vi "ADC Data capture and Process Original.vi"(0 "ADC Output Read Method":T2(ring)=enum."Read .dat file", 1 "Select the Tab to project":T1(ring)=enum."ADC Sine", 2 "ADC Input":enum16{"Sine Wave", "Ramp / Triangle"}(ring), 3 "No.of samples(SNR)":i32=4096, 4 "Resolution":i32=12, 5 "active edge":i32(ring)=10280, 6 "Inputs for Dyanmic para":T9={"Fundamental Frequency"=100000.0, "Sampling Frequncy"=3999610.0, "No of Harmonics"=9, "Window"=enum."7 Term B-Harris", "Blackman (fundamental power) bins)"=1.0}, 7 "Samples per Channel":i32=4096 caption="No.of Samples(capture)", 8 "Oversampling":bool, 9 "Oversampling ratio":i32, 10 "Drop LSB":bool, 11 "Save data":T15, 12 "Waveform":i64[](array[numeric]), 13 "Path to Read":path=path "C/Users/a0230227/Desktop/save.dat", 14 "Start & Stop Bit":cluster{"Start":i32, "Stop":i32}={"Start"=40, "Stop"=4055}, 15 "length":i32=4096, 17 "Set_Freq":dbl=100017.0, 24 "path to save":T14={"Path to Save plot"=path "D/Tenor_176P/DYN_PAR_C004/DAT/D001_TEMPP30C_VDD1.2_VDDA3.3_16B_SE_ADCA__vicA_aggX_PLT_CAP_200821_1740_33.jpg", "Path to Raw Data plot"=path "D/Tenor_176P/DYN_PAR_C004/DAT/D001_TEMPP30C_VDD1.2_VDDA3.3_16B_SE_ADCA__vicA_aggX_RAW_DAT_200821_1740_33.csv"}) -> (18 "Min Max":T4, 19 "detected Throughput":dbl, 20 "output cluster":T7, 21 "Dynamic Parameters":T8, 22 "max code":ext, 23 "min code":ext, 25 "Valid Capture":bool)   [LabVIEW 2021] (continued)
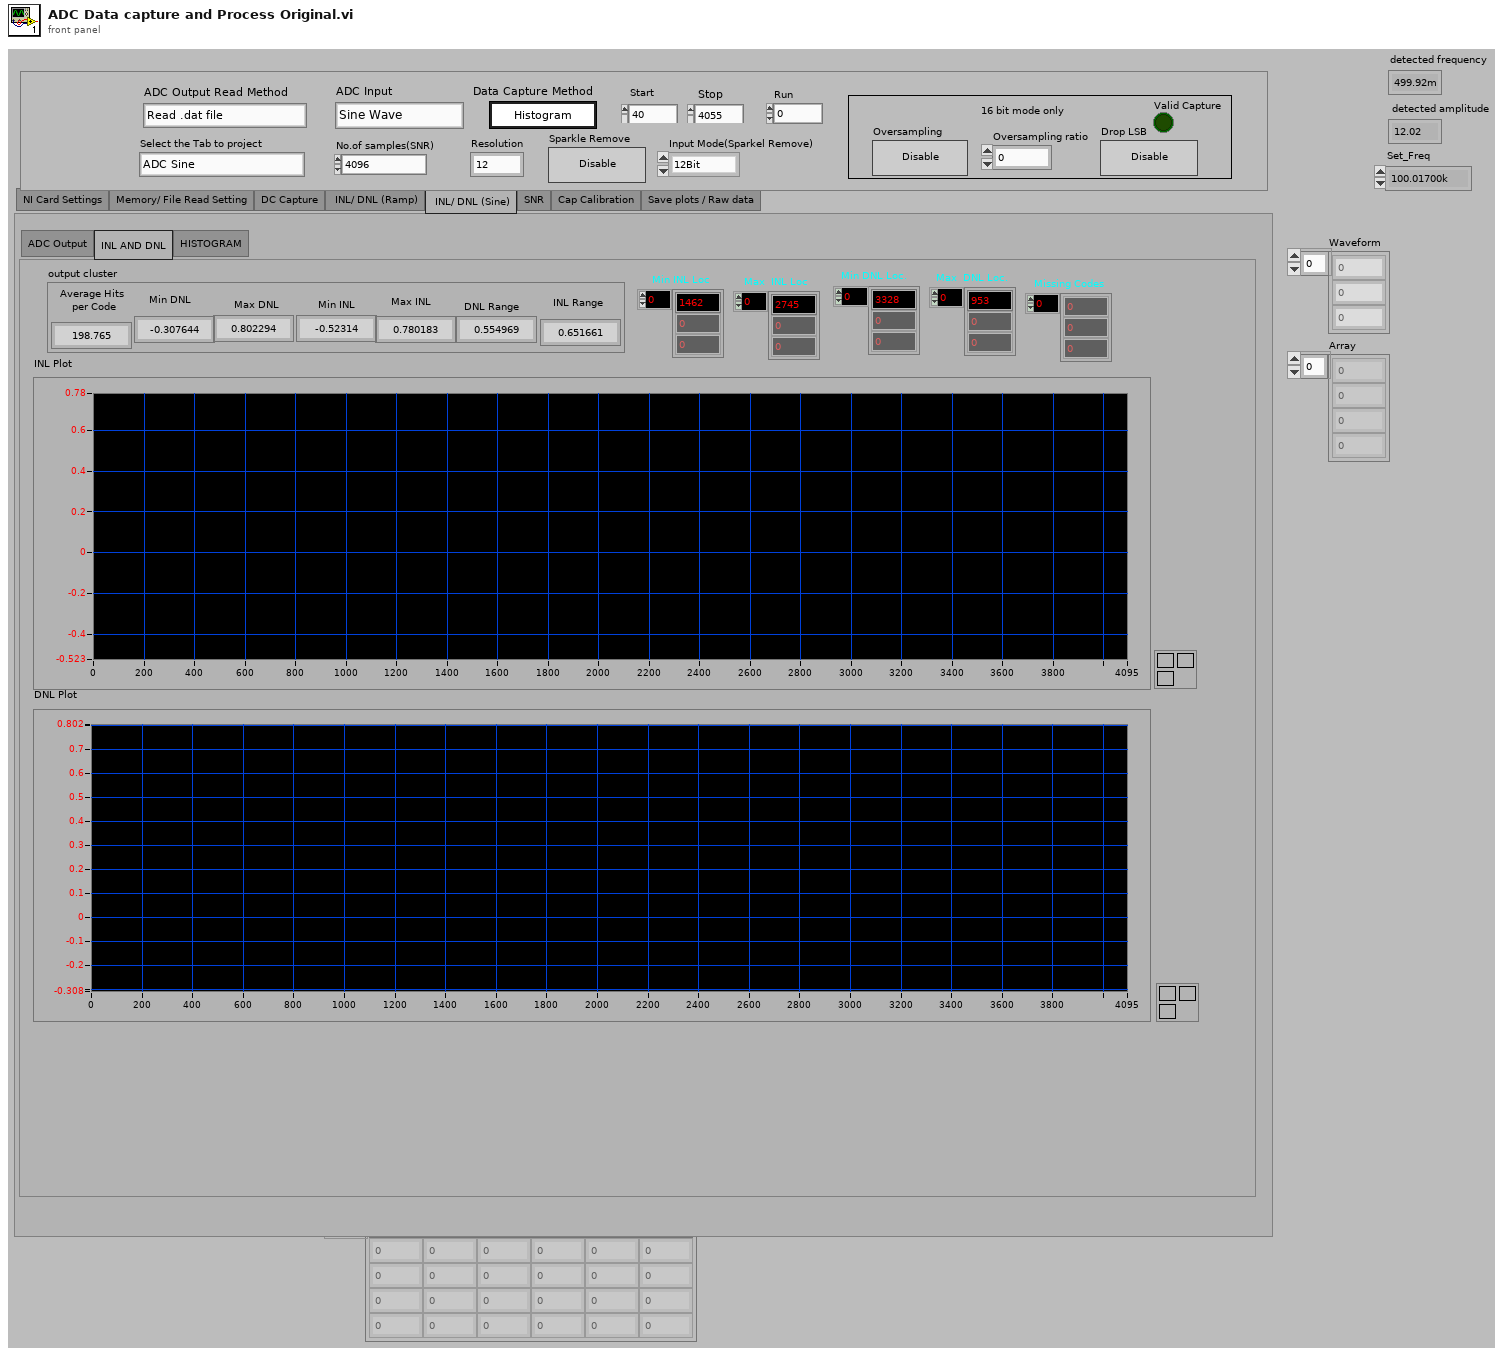
[diagram p1: front panel]
types:
  T1 = enum32{"NI Card Settings", "Memory Read Setting", "DC Capture", "ADC Ramp", "ADC Sine", "SNR", "Cap Calibration"}
  T2 = enum32{"Read from Memory", "Read .dat file", "NI Card Capture", "None"}
  T3 = enum32{"NI Card Settings", "Memory/ File Read Setting", "DC Capture", " INL/ DNL (Ramp)", " INL/ DNL (Sine)", "SNR", "Cap Calibration", "Save plots / Raw data"}
  T4 = cluster{"Min":dbl, "Max":dbl, "delta":dbl, "Average Code":dbl, "Standard Deviation":dbl}
  T5 = cluster{"Min INL":dbl, "Max INL":dbl, "Min DNL":dbl, "Max DNL":dbl, "INL Range":dbl, "DNL Range":dbl, "Avg Hits/Code":dbl}
  T6 = enum32{"ADC Output", "TRIMMED DATA", "INL AND DNL", "HISTOGRAM"}
  T7 = cluster{"Average Hits \nper Code ":dbl, "Min DNL":dbl, "Min INL":dbl, "Max INL":dbl, "Max DNL":dbl, "DNL Range":dbl, "INL Range":dbl}
  T8 = cluster{"SNR":dbl, "SNRD":dbl, "THD":dbl, "ENOB (SNRD)":dbl, "SFDR":dbl, "ENOB (SNR)":dbl, "Noise Power":dbl, "Signal power":dbl}
  T9 = cluster{"Fundamental Frequency":dbl, "Sampling Frequncy":dbl, "No of Harmonics":u8, "Window":enum16{"None ", "Hanning", "Hamming", "Blackman-Harris", "Exact Blackman", "Blackman", "Flat Top", "4 Term B-Harris ", "7 Term B-Harris"}, "Blackman (fundamental power) bins)":dbl}
  T10 = enum32{"ADC Output", "FFT Magnitude plot", " FFT plot"}
  T11 = cluster{"Ideal Power Bin":dbl, "Actual Power Bin":dbl, "Signal Strength (dB)":dbl}
  T12 = cluster{"ADC Reference(V)":dbl, "Bin Width":dbl, "PSRR/ CMRR  ":bool}
  T13 = cluster{"Fundamental Frequnecy (Calculated)":dbl, "Harmonic Frequencies":dbl[], "Harmonic Amplitudes":dbl[]}
  T14 = cluster{"Path to Save plot":path, "Path to Raw Data plot":path}
  T15 = cluster{"Save INL/DNL Plot(Ramp)":bool, "Save SNR Plot":bool, "Save INL/DNL Plot(Sine)":bool, "Save INL/DNL Raw Data(Ramp)":bool, "Save SNR Raw Data":bool, "Save INL/DNL Raw Data(Sine)":bool, "Save DC Raw data":bool, "Save  Raw Data(Sine)":bool}
  T16 = enum16{"Initialize", "Read output", "Post process", "Cap Calib", "Save data", "Exit"}
  T17 = cluster{"Average Hits \nper Code ":dbl, "Min\nDNL":dbl, dbl, dbl, "Max\nDNL":dbl, dbl, dbl}
  T18 = enum16{"None ", "Hanning", "Hamming", "Blackman-Harris", "Exact Blackman", "Blackman", "Flat Top", "4 Term B-Harris ", "7 Term B-Harris"}
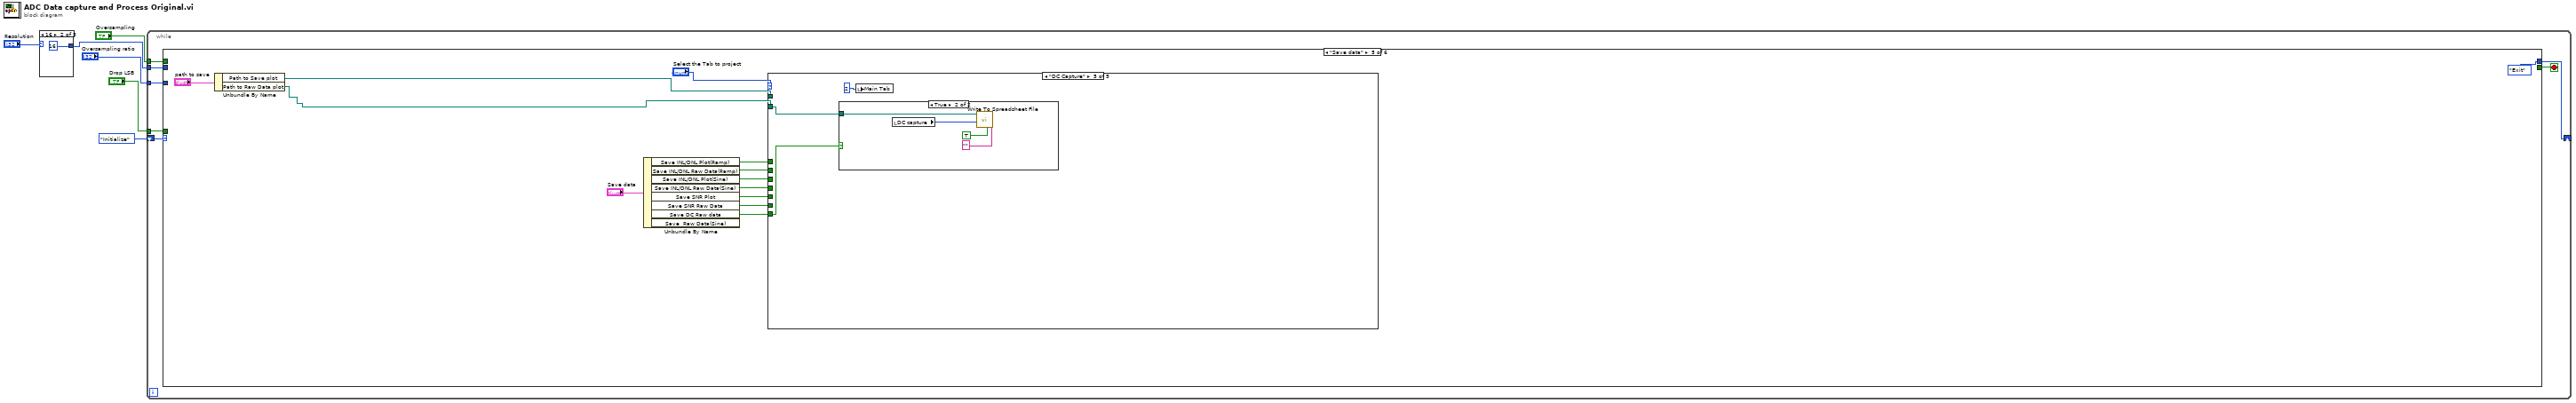
[diagram p0: block diagram]
diagram:
  n1 = case shown="16" "Resolution" {
    tunnel: [18 16 14 12 10] -> w5
    frame 18 {
    }
    frame 16 {
    }
    frame 14, Default {
    }
    frame 12 {
    }
    frame 10 {
    }
  }
  n2 = while {
    shift-right: [w17] -> _
    shift-left: T16."Initialize" -> [w18]
    tunnel: w5 -> [w15]
    tunnel: "Oversampling" -> [w14]
    tunnel: "Drop LSB" -> [w13]
    tunnel: "Oversampling ratio" -> [w12]
    stop <- w16 stop-if-true
    n3 = case shown="\"Save data\"" w18 {
      tunnel: [T16."Read output" w41 w104 T16."Save data" T16."Exit" _] -> w17
      tunnel: [_ _ _ _ _ TRUE] -> w16
      tunnel: w15 -> [_ _ w111 _ _ _]
      tunnel: w14 -> [_ _ w101 _ _ _]
      tunnel: w13 -> [_ _ w103 _ _ _]
      tunnel: w12 -> [_ _ w102 _ _ _]
      frame "Initialize", Default {
        n4 = local read "No.of samples(SNR)"() -> (w19:i32)
        n5 = local write "Samples per Channel"(w19) -> ()
      }
      frame "Read output" {
        w26 = waveform(i64) {"t0"=timestamp(0 s since 1904-01-01), "dt"=1.0, "Y"=[]}  # waveform
        n6 = case shown="\"NI Card Capture\", Default" "ADC Output Read Method" {
          tunnel: [w51 _ w70 "Waveform"] -> w27
          tunnel: [T16."Post process" _ T16."Post process" T16."Post process"] -> w41
          frame "Read .dat file" {
            w50 = 0  # index
            w56 = 8192 ("index")
            w61 = 1 ("index")
            n7 = call-poly <vilib>:"Read From Spreadsheet File.vi"("delimiter (\\t)"="Delimiter (\\t)", "file path (dialog if empty)"="Path to Read") -> ("all rows"=w63:i64[][])  [unwired: 5 in, 4 out]
            n8 = Index Array(array=w63, index (col)=0 ("disabled index (col)")) -> (element=w54:i64[])  [unwired: 1 in]
            n9 = Split 1D Array(array=w54, index=w61) -> (second subarray=w52:i64[])  [unwired: 1 out]
            n10 = Multiply(x=w56, y=1) -> (x*y=w59:i32)
            n11 = Multiply(x=2 ("y"), y=w56) -> (x*y=w57:i32)
            n12 = Multiply(x=w56, y=3) -> ()  [unwired: 1 out]
            n13 = Array Subset(array=w52, index=w61, length=w56) -> ()  [unwired: 1 out]
            n14 = Array Subset(array=w52, index=w59, length=w56) -> ()  [unwired: 1 out]
            n15 = Array Subset(array=w52, index=w57, length=w56) -> ()  [unwired: 1 out]
            n16 = Array Subset(array=w52, index=w50, length="length") -> (w51:i64[])
          }
          frame "None" {
          }
          frame "NI Card Capture", Default {
            n17 = case shown="\"Ramp / Triangle\"" "ADC Input" {
              tunnel: "Port" -> [w87 w98]
              tunnel: "Source" -> [w86 w97]
              tunnel: "Rate" -> [w85 w96]
              tunnel: "Timeout" -> [w84 w95]
              tunnel: [_ w93] -> w69
              tunnel: [w80 w94] -> w70
              tunnel: "No.of samples(SNR)" -> [w83 w92]
              tunnel: "Samples per Channel" -> [w81 w91]
              tunnel: "Sparkle Remove" -> [w79 _]
              tunnel: "active edge" -> [w78 w89]
              frame "Sine Wave", Default {
                n18 = call "DATA_CAPTURE_SNR.vi"("Port"=w87, "Source"=w86, "No. of samples to process"=w83, "Samples per Channel"=w81, "Rate"=w85, "active edge"=w78, "timeout"=w84, "Histogram Capture Method SNR"=w79, "NI card Cont/Single Capture"=FALSE ("Histogram Capture Method SNR")) -> ("Waveform"=w80:u32[])  [unwired: 5 in, 5 out]
              }
              frame "Ramp / Triangle" {
                n19 = call "DATA_CAPTURE_SNR.vi"("Port"=w98, "Source"=w97, "No. of samples to process"=w92, "Samples per Channel"=w91, "Rate"=w96, "active edge"=w89, "timeout"=w95, "Histogram Capture Method SNR"=FALSE, "NI card Cont/Single Capture"=FALSE ("Histogram Capture Method SNR")) -> ("Waveform"=w94:u32[], "Trimmed Wave"=w93:u32[])  [unwired: 5 in, 4 out]
              }
            }
            "Trimmed Wave" <- w69
          }
          frame "Read from Memory" {
          }
        }
        "Ramp Waveform" <- w27
        "Sine Waveform" <- w27
        "Read Data from Device" <- w27
        "Captured Data" <- w27
        "DC capture" <- w27
        n20 = Bundle By Name(cluster=w26, "Y"=w27) -> (w25:waveform(i64))
        n21 = Array Size(array=w27) -> (size(s)=w37:i32)
        n22 = Array Max & Min(array=w27) -> (max value=→"max code":i64, min value=→"min code":i64)  [unwired: 2 out]
        n23 = Decrement(x=w37) -> (x-1=w36:i32)
        n24 = call-poly <vilib>:"Extract Single Tone Information.vi"("time signal in"=w25) -> ("detected amplitude"=→"detected amplitude":dbl, "detected frequency"=w22:dbl)  [unwired: 5 in, 4 out]
        "detected frequency" <- w22
        n25 = for {
          N: w36 -> [_]
          tunnel: w27 -> [w48]
          tunnel: [w42] -> w34 mode=indexing
          i -> [w46]
          n26 = Increment(x=w46) -> (x+1=w47:i32)
          n27 = Index Array(array=w48, index=w46) -> (element=w44:i64)
          n28 = Index Array(array=w48, index=w47) -> (element=w45:i64)
          n29 = Subtract(x=w45, y=w44) -> (x-y=w43:i64)
          n30 = Absolute Value(x=w43) -> (abs(x)=w42:i64)
        }
        n31 = Divide(x="Set_Freq", y=w22) -> (x/y=→"detected Throughput":dbl)
        n32 = Add Array Elements(numeric array=w34) -> (sum=w32:i64)
        n33 = Array Max & Min(array=w34) -> (max value=w29:i64)  [unwired: 3 out]
        n34 = Array Size(array=w34) -> (size(s)=w31:i32)
        n35 = Divide(x=w32, y=w31) -> (x/y=w33:dbl)
        n36 = Multiply(x=2.0, y=w33) -> (x*y=w28:dbl)
        n37 = Less?(x=w29, y=w28) -> (x < y?=→"Valid Capture":bool)
      }
      frame "Post process" {
        n38 = local read "Select the Tab to project"() -> (w117:T1)
        n39 = local read "Read Data from Device"() -> (w108:dbl[])
        n40 = local read "No.of samples(SNR)"() -> (w110:i32)
        n41 = Equal?(x=w117, y=T1."Cap Calibration" ("Select the Tab to project")) -> (x = y?=w118:bool)
        n42 = Unbundle By Name("Start & Stop Bit") -> ("Start"=w113:i32, "Stop"=w112:i32)
        n43 = Select(t=T1."ADC Sine" ("Select the Tab to project"), s=w118, f=w117) -> (s? t:f=w116:T1)
        n44 = case shown="\"DC Capture\", Default" w116 {
          tunnel: w108 -> [w123 w239 w311 w376]
          tunnel: "Data Capture Method" -> [w120 w237 w344 _]
          tunnel: w113 -> [_ w236 w343 _]
          tunnel: w112 -> [_ w235 w342 _]
          tunnel: w111 -> [_ w238 w341 w375]
          tunnel: w110 -> [_ _ _ w377]
          tunnel: [_ w234 w329 _] -> w109
          tunnel: [T16."Save data" T16."Save data" T16."Cap Calib" T16."Save data"] -> w104
          tunnel: w101 -> [_ _ w308 w373]
          tunnel: w103 -> [_ _ w307 w372]
          tunnel: w102 -> [_ _ w309 w371]
          frame "DC Capture", Default {
            n45 = property on="Raw Data CH2" class="Arr (strict)"("Visible"="CH Swtich (To see other CH O/P)") -> ()  [unwired: 2 in, 2 out]
            n46 = property on="Standard Deviation (CH2)" class="DigNum (strict)"("Visible"="CH Swtich (To see other CH O/P)") -> ()  [unwired: 2 in, 2 out]
            n47 = property on="Raw Data CH1" class="Arr (strict)"("Visible"="CH Swtich (To see other CH O/P)") -> ()  [unwired: 2 in, 2 out]
            n48 = property on="Average Code (CH2)" class="DigNum (strict)"("Visible"="CH Swtich (To see other CH O/P)") -> ()  [unwired: 2 in, 2 out]
            n49 = case shown="False" w120 {
              tunnel: w123 -> [w126 w194]
              tunnel: "CH Swtich (To see other CH O/P)" -> [w125 _]
              tunnel: [w124 w180] -> w119
              frame False {
                n50 = case shown="True" w125 {
                  tunnel: w126 -> [w131 w168]
                  tunnel: [w127 w160] -> w124
                  frame True {
                    w137 = 10 ("index")
                    w150 = 10 ("index")
                    n51 = Decimate 1D Array(w131) -> (w147:dbl[], w138:dbl[])
                    "Raw Data CH2" <- w147
                    "Raw Data CH1" <- w138
                    n52 = Split 1D Array(array=w147, index=w150) -> (second subarray=w149:dbl[])  [unwired: 1 out]
                    n53 = Split 1D Array(array=w138, index=w137) -> (second subarray=w146:dbl[])  [unwired: 1 out]
                    n54 = Array Size(array=w149) -> (size(s)=w151:i32)
                    n55 = Array Size(array=w146) -> (size(s)=w145:i32)
                    n56 = Subtract(x=w151, y=w150) -> (x-y=w154:i32)
                    n57 = Subtract(x=w145, y=w137) -> (x-y=w135:i32)
                    n58 = Split 1D Array(array=w149, index=w154) -> (first subarray=w153:dbl[])  [unwired: 1 out]
                    n59 = Split 1D Array(array=w146, index=w135) -> (first subarray=w143:dbl[])  [unwired: 1 out]
                    n60 = Array Size(array=w153) -> (size(s)=w152:i32)
                    n61 = Array Size(array=w143) -> (size(s)=w144:i32)
                    n62 = To Double Precision Float(number=w153) -> (double precision float=w155:dbl[])
                    n63 = To Double Precision Float(number=w143) -> (double precision float=w134:dbl[])
                    n64 = Add Array Elements(numeric array=w155) -> (sum=w159:dbl)
                    n65 = Add Array Elements(numeric array=w134) -> (sum=w139:dbl)
                    n66 = Divide(x=w159, y=w152) -> (x/y=w132:dbl)
                    "Average Code (CH2)" <- w132
                    n67 = Divide(x=w139, y=w144) -> (x/y=w129:dbl)
                    n68 = Subtract(x=w155, y=w132) -> (x-y=w158:dbl[])
                    n69 = Subtract(x=w134, y=w129) -> (x-y=w140:dbl[])
                    n70 = Square(x=w158) -> (x^2=w157:dbl[])
                    n71 = Square(x=w140) -> (x^2=w141:dbl[])
                    n72 = Add Array Elements(numeric array=w157) -> (sum=w156:dbl)
                    n73 = Add Array Elements(numeric array=w141) -> (sum=w142:dbl)
                    n74 = Divide(x=w156, y=w152) -> (x/y=w148:dbl)
                    n75 = Divide(x=w142, y=w144) -> (x/y=w136:dbl)
                    n76 = Square Root(x=w148) -> (sqrt(x)=→"Standard Deviation (CH2)":dbl)
                    n77 = Square Root(x=w136) -> (sqrt(x)=w128:dbl)
                    n78 = local read "Min Max"() -> (w130:T4)
                    n79 = Bundle By Name(cluster=w130, "Average Code"=w129, "Standard Deviation"=w128) -> (w127:T4)
                  }
                  frame False {
                    w172 = 10 ("index")
                    n80 = Split 1D Array(array=w168, index=w172) -> (second subarray=w179:dbl[])  [unwired: 1 out]
                    n81 = Array Size(array=w179) -> (size(s)=w178:i32)
                    n82 = Subtract(x=w178, y=w172) -> (x-y=w170:i32)
                    n83 = Split 1D Array(array=w179, index=w170) -> (first subarray=w167:dbl[])  [unwired: 1 out]
                    n84 = Array Size(array=w167) -> (size(s)=w177:i32)
                    n85 = To Double Precision Float(number=w167) -> (double precision float=w169:dbl[])
                    n86 = Add Array Elements(numeric array=w169) -> (sum=w173:dbl)
                    n87 = Divide(x=w173, y=w177) -> (x/y=w162:dbl)
                    n88 = Subtract(x=w169, y=w162) -> (x-y=w174:dbl[])
                    n89 = Square(x=w174) -> (x^2=w175:dbl[])
                    n90 = Add Array Elements(numeric array=w175) -> (sum=w176:dbl)
                    n91 = Divide(x=w176, y=w177) -> (x/y=w171:dbl)
                    n92 = Array Max & Min(array=w167) -> (max value=w164:dbl, min value=w163:dbl)  [unwired: 2 out]
                    n93 = local read "Min Max"() -> (w166:T4)
                    n94 = Subtract(x=w164, y=w163) -> (x-y=w165:dbl)
                    n95 = Square Root(x=w171) -> (sqrt(x)=w161:dbl)
                    n96 = Bundle By Name(cluster=w166, "Standard Deviation"=w161, "Average Code"=w162, "Max"=w164, "Min"=w163, "delta"=w165) -> (w160:T4)
                  }
                }
              }
              frame True {
                n97 = for {
                  tunnel: w194 -> [w227] mode=indexing
                  shift-right: [w231] -> w203
                  shift-left: 0.0 ("x*y") -> [w232]
                  tunnel: w194 -> [w230]
                  tunnel: [w229] -> w202
                  shift-right: [w218] -> _
                  shift-left: TRUE ("x != 0?") -> [w225]
                  shift-right: [w221] -> w185
                  shift-left: i32[] [] -> [w222]
                  i -> [w224]
                  n98 = Add Array Elements(numeric array=w230) -> (sum=w229:dbl)
                  n99 = Not Equal To 0?(x=w227) -> (x != 0?=w226:bool)
                  n100 = Multiply(x=w227, y=w224) -> (x*y=w228:dbl)
                  n101 = Build Array (concatenate)(w222, w224) -> (w223:i32[])
                  n102 = And(x=w225, y=w226) -> (x .and. y?=w220:bool)
                  n103 = Add(x=w232, y=w228) -> (x+y=w231:dbl)
                  n104 = Select(t=w223, s=w220, f=w222) -> (s? t:f=w221:i32[])
                  n105 = Select(t=FALSE ("x != 0?"), s=w220, f=TRUE ("x != 0?")) -> (s? t:f=w218:bool)
                }
                n106 = Divide(x=w203, y=w202) -> (x/y=w181:dbl)
                n107 = Array Size(array=w185) -> (size(s)=w183:i32)
                n108 = Index Array(array=w185, index=0) -> (element=w186:i32)
                n109 = Split 1D Array(array=w194, index=w186) -> (second subarray=w189:dbl[])  [unwired: 1 out]
                n110 = Subtract(x=w183, y=15 ("x")) -> (x-y=w182:i32)
                n111 = Array Max & Min(array=w189) -> (max index (indices)=w197:i32)  [unwired: 3 out]
                n112 = Greater?(x=w197, y=w182) -> (0:w198:bool)
                n113 = case shown="True" w198 {
                  tunnel: w197 -> [w206 w213]
                  tunnel: [w205 w213] -> w193
                  tunnel: 10 ("y") -> [w210 w212]
                  tunnel: w189 -> [w209 w216]
                  tunnel: [w206 w215] -> w192
                  tunnel: [_ w211] -> w187
                  frame True {
                    n114 = Subtract(x=w206, y=w210) -> (x-y=w207:i32)
                    n115 = Split 1D Array(array=w209, index=w207) -> (first subarray=w208:dbl[])  [unwired: 1 out]
                    n116 = Array Max & Min(array=w208) -> (max index (indices)=w205:i32)  [unwired: 3 out]
                  }
                  frame False {
                    n117 = Add(x=w213, y=w212) -> (x+y=w211:i32)
                    n118 = Split 1D Array(array=w216, index=w211) -> (second subarray=w214:dbl[])  [unwired: 1 out]
                    n119 = Array Max & Min(array=w214) -> (max index (indices)=w215:i32)  [unwired: 3 out]
                  }
                }
                n120 = Add(x=w186, y=w193) -> (x+y=w190:i32)
                n121 = Compound Arithmetic op=ADD(w186, w192, w187) -> (w191:i32)
                n122 = Subtract(x=w191, y=w190) -> (x-y=w196:i32)
                n123 = local read "Min Max"() -> (w201:T4)
                n124 = Bundle By Name(cluster=w201, "Average Code"=w181, "Min"=w190, "Max"=w191, "delta"=w196) -> (w180:T4)
              }
            }
            "Min Max" <- w119
          }
          frame "ADC Ramp" {
            n125 = stacked-sequence {
              seq-local: [w241 _ _] -> [_ w265 _]
              seq-local: [_ w261 _] -> [_ _ w291]
              seq-local: [_ w260 _] -> [_ _ w290]
              seq-local: [_ w259 _] -> [_ _ w279]
              seq-local: [w242 _ _] -> [_ w258 _]
              tunnel: w239 -> [w244 _ _]
              tunnel: w238 -> [w246 _ _]
              tunnel: w237 -> [w245 _ _]
              tunnel: w236 -> [_ w264 _]
              tunnel: w235 -> [_ w263 _]
              tunnel: [w241 _ _] -> w234
              frame #0 {
                n126 = local read "Trimmed Wave"() -> (w240:u32[])
                n127 = Scale By Power Of 2(n=w246, x=ext 1.0) -> (x*2^n=w242:ext)
                n128 = Initialize Array(0 ("element"), w242) -> (w250:i32[])
                n129 = for {
                  shift-right: [w253] -> w243
                  shift-left: w250 -> [w254]
                  tunnel: 0.0 -> [w252]
                  tunnel: w240 -> [w251] mode=indexing
                  n130 = Subtract(x=w251, y=w252) -> (x-y=w255:dbl)
                  n131 = in-place {
                    n132 = in-place-array #1(w254, w255) -> (w257:i32)
                    n133 = Increment(x=w257) -> (x+1=w256:i32)
                    n134 = in-place-array #1(w256) -> (w253:i32[])  [unwired: 1 out]
                  }
                }
                n135 = Select(t=w244, s=w245, f=w243) -> (s? t:f=w241:dbl[])
                "Histogram waveform" <- w241
              }
              frame #1 {
                n136 = Subtract(x=w263, y=w264) -> (x-y=w266:i32)
                n137 = Split 1D Array(array=w265, index=w264) -> (second subarray=w273:dbl[])  [unwired: 1 out]
                n138 = Split 1D Array(array=w273, index=w266) -> (first subarray=w267:dbl[])  [unwired: 1 out]
                n139 = Add Array Elements(numeric array=w267) -> (sum=w270:dbl)
                n140 = Array Size(array=w267) -> (size(s)=w269:i32)
                n141 = Divide(x=w270, y=w269) -> (x/y=w259:dbl)
                n142 = Initialize Array(w259, w258) -> (w268:dbl[])
                n143 = Replace Array Subset(array=w268, new element=w267, index=w264) -> (w272:dbl[])
                n144 = Divide(x=w272, y=w259) -> (x/y=w271:dbl[])
                n145 = Decrement(x=w271) -> (x-1=w261:dbl[])
                "DNL_Ramp" <- w261
                n146 = for {
                  shift-right: [w275] -> _
                  shift-left: 0.0 ("x") -> [w276]
                  tunnel: [w275] -> w260 mode=indexing
                  tunnel: w261 -> [w274] mode=indexing
                  n147 = Add(x=w276, y=w274) -> (x+y=w275:dbl)
                }
                "INL_Ramp" <- w260
              }
              frame #2 {
                n148 = Array Max & Min(array=w291) -> (max value=w282:dbl, min value=w283:dbl)  [unwired: 2 out]
                n149 = Array Max & Min(array=w290) -> (max value=w284:dbl, min value=w285:dbl)  [unwired: 2 out]
                n150 = Subtract(x=w282, y=w283) -> (x-y=w287:dbl)
                n151 = Subtract(x=w284, y=w285) -> (x-y=w288:dbl)
                n152 = local read "Static Parameters (Ramp)"() -> (w278:T5)
                n153 = Divide(x=w287, y=2.0) -> (x/y=w280:dbl)
                n154 = Divide(x=w288, y=2.0) -> (x/y=w281:dbl)
                n155 = disable-structure shown="Enabled" {
                  disable-tunnel: w285 -> [w306 _]
                  disable-tunnel: w284 -> [w305 _]
                  disable-tunnel: w283 -> [w304 _]
                  disable-tunnel: w282 -> [w303 _]
                  disable-tunnel: w281 -> [w294 _]
                  disable-tunnel: w280 -> [w293 _]
                  disable-tunnel: w279 -> [w292 _]
                  frame Disabled {
                    n156 = Increment(x="Run") -> (x+1=w295:dbl)
                    n157 = local write "Run"(w295) -> ()
                    n158 = Build Array(w295, w306, w305, w304, w303, w294, w293, w292) -> (w302:dbl[])
                    n159 = call-poly <vilib>:"Write To Spreadsheet File.vi"("delimiter (\\t)"="," ("delimiter (\\t)"), "transpose? (no:F)"=FALSE, "format (%.3f)"="%.4f", "append to file? (new file:F)"=TRUE, "1D data"=w302, "file path (dialog if empty)"=path "D:/FALCON/ADC/Raw_Data/runtorun.csv") -> ()  [unwired: 2 in, 1 out]
                  }
                  frame Enabled {
                  }
                }
                n160 = Bundle By Name(cluster=w278, "Max INL"=w284, "Min INL"=w285, "Max DNL"=w282, "Min DNL"=w283, "INL Range"=w281, "DNL Range"=w280, "Avg Hits/Code"=w279) -> (→"Static Parameters (Ramp)":T5)
              }
            }
          }
          frame "ADC Sine" {
            n161 = case shown="True" w308 {
              tunnel: w311 -> [w346 w354]
              tunnel: [w347 w352] -> w310
              tunnel: w309 -> [_ w353]
              tunnel: w307 -> [w345 _]
              frame False {
                n162 = case shown="True" w345 {
                  tunnel: w346 -> [w348 w350]
                  tunnel: [w348 w349] -> w347
                  frame False {
                  }
                  frame True {
                    n163 = Divide(x=w350, y=2.0) -> (x/y=w349:dbl[])
                  }
                }
              }
              frame True {
                n164 = Array Size(array=w354) -> (size(s)=w356:i32)
                n165 = Divide(x=w356, y=w353) -> (x/y=w355:dbl)
                n166 = for {
                  N: w355 -> [_]
                  tunnel: w354 -> [w363]
                  tunnel: w353 -> [w358]
                  tunnel: [w357] -> w352 mode=indexing
                  i -> [w362]
                  n167 = Multiply(x=w358, y=w362) -> (x*y=w361:i32)
                  n168 = Array Subset(array=w363, index=w361, length=w358) -> (w360:dbl[])
                  n169 = Add Array Elements(numeric array=w360) -> (sum=w359:dbl)
                  n170 = Divide(x=w359, y=w358) -> (x/y=w357:dbl)
                }
              }
            }
            n171 = call "Sinewave_Linearity_trial_F027.vi"("Array"=w310, "Histogram Capture Method"=w344, "L code"=w343, "UCode"=w342, "Resolution"=w341, "Histogram: h(x)"=w310) -> ("Average Hits \nper Code"=w319:dbl, "Max\nDNL"=w315:dbl, "Min\nDNL"=w318:dbl, "Missing Codes"=→"Missing Codes":i32[], "Max  DNL Loc."=→"Max  DNL Loc.":i32[], "Min DNL Loc."=→"Min DNL Loc.":i32[], "Max  INL Loc"=→"Max  INL Loc":i32[], "Min INL Loc"=→"Min INL Loc":i32[], "Histogram Plot"=w331:dbl[][], "DNL Plot"=w327:dbl[], "INL Plot"=w320:dbl[])  [unwired: 1 in, 2 out]
            "Histogram Plot" <- w331
            "DNL Plot" <- w327
            "INL Plot" <- w320
            n172 = for {
              tunnel: w327 -> [w370] mode=indexing
              tunnel: [w366] -> w326 mode=indexing
              shift-right: [w365] -> _
              shift-left: 16384 ("f") -> [w364]
              i -> [w367]
              n173 = Increment(x=w364) -> (x+1=w365:i32)
              n174 = Greater?(x=w370, y=0.9) -> (0:w368:bool)
              n175 = Select(t=w367, s=w368, f=w364) -> (s? t:f=w366:i32)
            }
            n176 = Subtract(x=w315, y=w318) -> (x-y=w338:dbl)
            n177 = Array Max & Min(array=w320) -> (max value=w316:dbl, min value=w317:dbl)  [unwired: 2 out]
            n178 = Index Array(array=w331, index (col)=1 ("disabled index (col)")) -> (element=w329:dbl[])  [unwired: 1 in]
            n179 = Subtract(x=w316, y=w317) -> (x-y=w340:dbl)
            n180 = Divide(x=w338, y=2.0) -> (x/y=w314:dbl)
            n181 = Divide(x=w340, y=2.0) -> (x/y=w313:dbl)
            n182 = Bundle("Average Hits \nper Code"=w319, "Min\nDNL"=w318, w317, w316, "Max\nDNL"=w315, w314, w313) -> (→"output cluster":T17)  [unwired: 1 in]
            n183 = Sort 1D Array(array=w326) -> (sorted array=w322:i32[])
            n184 = Search 1D Array(1D array=w322, element=16384) -> (index of element=w323:i32)  [unwired: 1 in]
            n185 = Array Subset(array=w322, length=w323) -> (→"Array":i32[])  [unwired: 1 in]
          }
          frame "SNR" {
            n186 = stacked-sequence {
              seq-local: [w398 _ _] -> [_ w459 _]
              seq-local: [w397 _ _] -> [_ _ w484]
              seq-local: [w391 _ _] -> [_ _ w487]
              seq-local: [w390 _ _] -> [_ _ w483]
              seq-local: [w389 _ _] -> [_ _ w482]
              tunnel: w377 -> [w410 _ w485]
              tunnel: w376 -> [w392 _ _]
              tunnel: w375 -> [w394 _ _]
              tunnel: w373 -> [w381 _ _]
              tunnel: w372 -> [w380 _ _]
              tunnel: w371 -> [w379 _ _]
              frame #0 {
                n187 = Unbundle By Name("PSRR/CMRR Input") -> ("ADC Reference(V)"=w393:dbl, "PSRR/ CMRR"=w389:bool)
                n188 = case shown="True" w389 {
                  tunnel: 1.0 ("x") -> [_ w445]
                  tunnel: w394 -> [_ w444]
                  tunnel: w393 -> [_ w442]
                  tunnel: w392 -> [w438 w440]
                  tunnel: [w438 w439] -> w383
                  frame False {
                  }
                  frame True {
                    n189 = Scale By Power Of 2(n=w444, x=w445) -> (x*2^n=w443:dbl)
                    n190 = Divide(x=w442, y=w443) -> (x/y=w441:dbl)
                    n191 = Multiply(x=w440, y=w441) -> (x*y=w439:dbl[])
                  }
                }
                n192 = case shown="True" w381 {
                  tunnel: w383 -> [w420 w428]
                  tunnel: [w421 w426] -> w382
                  tunnel: w379 -> [_ w427]
                  tunnel: w380 -> [w419 _]
                  frame False {
                    n193 = case shown="True" w419 {
                      tunnel: w420 -> [w422 w424]
                      tunnel: [w422 w423] -> w421
                      frame False {
                      }
                      frame True {
                        n194 = Divide(x=w424, y=2.0) -> (x/y=w423:dbl[])
                      }
                    }
                  }
                  frame True {
                    n195 = Array Size(array=w428) -> (size(s)=w430:i32)
                    n196 = Divide(x=w430, y=w427) -> (x/y=w429:dbl)
                    n197 = for {
                      N: w429 -> [_]
                      tunnel: w428 -> [w437]
                      tunnel: w427 -> [w432]
                      tunnel: [w431] -> w426 mode=indexing
                      i -> [w436]
                      n198 = Multiply(x=w432, y=w436) -> (x*y=w435:i32)
                      n199 = Array Subset(array=w437, index=w435, length=w432) -> (w434:dbl[])
                      n200 = Add Array Elements(numeric array=w434) -> (sum=w433:dbl)
                      n201 = Divide(x=w433, y=w432) -> (x/y=w431:dbl)
                    }
                  }
                }
                n202 = Unbundle By Name("Inputs for Dyanmic para") -> ("Window"=w408:T18, "Sampling Frequncy"=w397:dbl, "Fundamental Frequency"=w391:dbl, "No of Harmonics"=w398:u8, "Blackman (fundamental power) bins)"=w407:dbl)
                n203 = Reciprocal(x=w397) -> (1/x=w412:dbl)
                n204 = call-poly <vilib>:"Scaled Time Domain Window.vi"("window"=w408, "X"=w382) -> ("Windowed X"=w416:dbl[])  [unwired: 7 in, 2 out]
                n205 = local read "Dynamic Parameters"() -> (w406:T8)
                n206 = call <vilib>:"Auto Power Spectrum.vi"("dt"=w412, "Signal (V)"=w416) -> ("Power Spectrum (V^2 rms)"=w411:dbl[])  [unwired: 1 out]
                n207 = Logarithm Base 10(1:w411) -> (0:w418:dbl[])
                n208 = call "Calculate_SNR_THD.vi"("Auto Power Spectrum"=w411, "frame size"=w410, "# harmonics"=w398, "window"=w408, "sampling rate"=w397, "fundamental frequency"=w391, "Blackman\n (fundamental power bins)"=w407) -> ("% THD"=w405:dbl, "ENOB(SNRD)"=w400:dbl, "% THD + Noise"=w378:dbl, "ENOB(SNR)"=w401:dbl, "Noise Power"=w404:dbl, "Fundamental frequency Calculated"=w386:dbl, "SNR"=w403:dbl, "Signal power"=w402:dbl, "Harmonic Amplitudes"=w413:dbl[], "Harmonic Frequencies"=w388:dbl[])  [unwired: 3 in]
                n209 = Bundle By Name(cluster=w406, "THD"=w405, "SNRD"=w378, "Noise Power"=w404, "SNR"=w403, "Signal power"=w402, "ENOB (SNR)"=w401, "ENOB (SNRD)"=w400) -> (→"Dynamic Parameters":T8)
                n210 = Logarithm Base 10(1:w413) -> (0:w415:dbl[])
                n211 = Multiply(x=10.0, y=w418) -> (x*y=w390:dbl[])
                "FFT Magnitude Plot (dB)" <- w390
                n212 = local read "Harmonic Details"() -> (w384:T13)
                n213 = Multiply(x=20, y=w415) -> (x*y=w387:dbl[])
                n214 = Bundle By Name(cluster=w384, "Fundamental Frequnecy (Calculated)"=w386, "Harmonic Frequencies"=w388, "Harmonic Amplitudes"=w387) -> (→"Harmonic Details":T13)
              }
              frame #1 {
                n215 = local read "Harmonic Details"() -> (w447:T13)
                n216 = Unbundle By Name(w447) -> ("Harmonic Amplitudes"=w446:dbl[])
                n217 = Decrement(x=w459) -> (x-1=w465:u8)
                n218 = Index Array(array=w446, index=0) -> (element=w461:dbl)
                n219 = Array Subset(array=w446, index=1, length=w465) -> (w463:dbl[])
                n220 = Array Max & Min(array=w463) -> (max value=w460:dbl)  [unwired: 3 out]
                n221 = local read "Dynamic Parameters"() -> (w458:T8)
                n222 = Subtract(x=w461, y=w460) -> (x-y=w457:dbl)
                n223 = Bundle By Name(cluster=w458, "SFDR"=w457) -> (w456:T8)
                n224 = local write "Dynamic Parameters"(w456) -> ()
                n225 = Unbundle By Name(w456) -> ("SNR"=w455:dbl, "SNRD"=w454:dbl, "THD"=w453:dbl, "SFDR"=w452:dbl, "ENOB (SNR)"=w451:dbl, "ENOB (SNRD)"=w450:dbl, "Noise Power"=w449:dbl, "Signal power"=w448:dbl)
                n226 = disable-structure shown="Disabled" {
                  disable-tunnel: w455 -> [w481 _]
                  disable-tunnel: w454 -> [w480 _]
                  disable-tunnel: w450 -> [w468 _]
                  disable-tunnel: w453 -> [w471 _]
                  disable-tunnel: w452 -> [w470 _]
                  disable-tunnel: w451 -> [w469 _]
                  disable-tunnel: w449 -> [w467 _]
                  disable-tunnel: w448 -> [w466 _]
                  frame Disabled {
                    n227 = local read "Run"() -> (w472:dbl)
                    n228 = Increment(x=w472) -> (x+1=w473:dbl)
                    n229 = local write "Run"(w473) -> ()
                    n230 = Build Array(w473, w481, w480, w471, w470, w469, w468, w467, w466) -> (w479:dbl[])
                    n231 = call-poly <vilib>:"Write To Spreadsheet File.vi"("delimiter (\\t)"="," ("delimiter (\\t)"), "transpose? (no:F)"=FALSE, "format (%.3f)"="%.4f", "append to file? (new file:F)"=TRUE, "1D data"=w479, "file path (dialog if empty)"=path "D:/FALCON/ADC/Raw_Data/runtorun.csv") -> ()  [unwired: 2 in, 1 out]
                  }
                  frame Enabled {
                  }
                }
              }
              frame #2 {
                n232 = local read "FFT Magnitude Plot (dB)"() -> (w494:dbl[])
                n233 = Array Size(array=w494) -> (size(s)=w493:i32)
                n234 = Divide(x=w484, y=2.0) -> (x/y=w491:dbl)
                n235 = for {
                  N: w493 -> [_]
                  tunnel: w494 -> [w537]
                  tunnel: [w532] -> w489 mode=indexing
                  tunnel: w493 -> [w535]
                  tunnel: w491 -> [w533]
                  tunnel: [w531] -> w490 mode=indexing
                  tunnel: [w531] -> w486
                  i -> [w536]
                  n236 = Divide(x=w536, y=w535) -> (x/y=w534:dbl)
                  n237 = Index Array(array=w537, index=w536) -> (element=w532:dbl)
                  n238 = Multiply(x=w534, y=w533) -> (x*y=w531:dbl)
                }
                n239 = case shown="True" w482 {
                  tunnel: w487 -> [_ w498]
                  tunnel: w486 -> [_ w499]
                  tunnel: w485 -> [_ w513]
                  tunnel: w484 -> [_ w501]
                  tunnel: w483 -> [_ w505]
                  frame False {
                  }
                  frame True {
                    n240 = Greater?(x=w498, y=w499) -> (0:w500:bool)
                    n241 = case shown="False" w500 {
                      tunnel: [w516 w517] -> w497
                      tunnel: w498 -> [w516 w523]
                      tunnel: w501 -> [_ w522]
                      tunnel: w499 -> [_ _]
                      tunnel: w498 -> [_ w521]
                      frame False {
                      }
                      frame True {
                        n242 = while {
                          tunnel: w522 -> [w530]
                          tunnel: w523 -> [w527]
                          shift-right: [w525] -> _
                          shift-left: w522 -> [w524]
                          shift-left: w522 -> [_]
                          tunnel: [w524] -> w520
                          i -> [w528]
                          stop <- w526 continue-if-true
                          n243 = Increment(x=w528) -> (x+1=w529:i32)
                          n244 = Multiply(x=w530, y=w529) -> (x*y=w525:dbl)
                          n245 = Greater?(x=w527, y=w525) -> (0:w526:bool)
                        }
                        n246 = Subtract(x=w520, y=w521) -> (x-y=w518:dbl)
                        n247 = Sign(1:w518) -> (0:w519:dbl)
                        n248 = Multiply(x=w518, y=w519) -> (x*y=w517:dbl)
                      }
                    }
                    n249 = Multiply(x=w513, y=w497) -> (x*y=w515:dbl)
                    n250 = local read "PSRR/CMRR Input"() -> (w511:T12)
                    n251 = Divide(x=w515, y=w501) -> (x/y=w514:dbl)
                    n252 = Unbundle By Name(w511) -> ("Bin Width"=w496:dbl)
                    n253 = To Long Integer(number=w514) -> (32bit integer=w510:i32)
                    n254 = Subtract(x=w510, y=w496) -> (x-y=w506:dbl)
                    n255 = Add(x=w510, y=w496) -> (x+y=w495:dbl)
                    n256 = Split 1D Array(array=w505, index=w495) -> (first subarray=w509:dbl[])  [unwired: 1 out]
                    n257 = Split 1D Array(array=w509, index=w506) -> (second subarray=w508:dbl[])  [unwired: 1 out]
                    n258 = Array Max & Min(array=w508) -> (max value=w504:dbl, max index (indices)=w507:i32)  [unwired: 2 out]
                    n259 = local read "PSRR/CMRR Output"() -> (w512:T11)
                    n260 = Add(x=w507, y=w506) -> (x+y=w503:dbl)
                    n261 = Bundle By Name(cluster=w512, "Ideal Power Bin"=w510, "Actual Power Bin"=w503, "Signal Strength (dB)"=w504) -> (→"PSRR/CMRR Output":T11)
                  }
                }
                n262 = Bundle(w490, w489) -> (→"FFT Plot":cluster{dbl[], dbl[]})  [unwired: 1 in]
              }
            }
          }
        }
        n263 = Build Array(w108, w109) -> (→"Raw_Histo":dbl[][])
      }
      frame "Cap Calib" {
        n264 = case shown="\"32\"" "Average Window" {
          tunnel: [8 16 32 64] -> w538
          frame "8", Default {
          }
          frame "16" {
          }
          frame "32" {
          }
          frame "64" {
          }
        }
        n265 = case shown="True" "Cap Calibration" {
          tunnel: w538 -> [_ w546]
          frame False {
          }
          frame True {
            n266 = local read "DNL Plot"() -> (w547:dbl[])
            n267 = local read "INL Plot"() -> (w548:dbl[])
            n268 = call "Cap_Calibration.vi"("INL"=w548, "DNL"=w547, "From File/ Waveform"="INL/DNL Values", "Select Channel"="Select Channel", "Average Window"=w546, "File path (DNL & INL)"="File path (DNL & INL)") -> ("ADC TEST 7"=→"ADC TEST 7":string, "ADC TEST 6"=→"ADC TEST 6":string, "ADC TEST 5"=→"ADC TEST 5":string, "Trim Coeff (Binary)"=→"Trim Coeff (Binary)":string[], "Trim Coeff (Integer)"=→"Trim Coeff (Integer)":dbl[])  [unwired: 1 in]
          }
        }
      }
      frame "Save data" {
        n269 = Unbundle By Name("path to save") -> ("Path to Save plot"=w557:path, "Path to Raw Data plot"=w558:path)
        n270 = Unbundle By Name("Save data") -> ("Save INL/DNL Plot(Ramp)"=w566:bool, "Save INL/DNL Raw Data(Ramp)"=w565:bool, "Save INL/DNL Plot(Sine)"=w564:bool, "Save INL/DNL Raw Data(Sine)"=w563:bool, "Save SNR Plot"=w562:bool, "Save SNR Raw Data"=w561:bool, "Save DC Raw data"=w559:bool)  [unwired: 1 out]
        n271 = case shown="\"DC Capture\"" "Select the Tab to project" {
          tunnel: w557 -> [w573 w592 w616 _ _]
          tunnel: w558 -> [w574 w593 w615 _ w632]
          tunnel: w566 -> [w571 _ _ _ _]
          tunnel: w565 -> [w570 _ _ _ _]
          tunnel: w564 -> [_ w590 _ _ _]
          tunnel: w563 -> [_ w589 _ _ _]
          tunnel: w562 -> [_ _ w613 _ _]
          tunnel: w561 -> [_ _ w612 _ _]
          tunnel: w559 -> [_ _ _ _ w631]
          frame "ADC Ramp" {
            n272 = case shown="True" w571 {
              tunnel: w573 -> [_ w575]
              frame False {
              }
              frame True {
                n273 = Current VI's Path() -> (path=w576:path)
                n274 = call "Take fron panel screenshot.vi"("VI path"=w576, "Image path"=w575, "Visible area only? (f)"=FALSE, "File type (.jpg)"=enum16{".bmp", ".png", ".jpg"}.".png") -> ()  [unwired: 4 in, 1 out]
              }
            }
            n275 = case shown="True" w570 {
              tunnel: w574 -> [_ w582]
              frame False {
              }
              frame True {
                w581 = "" ("delimiter (\\t)")
                w580 = TRUE ("transpose? (no:F)")
                n276 = local read "Histogram waveform"() -> (w585:dbl[])
                n277 = local read "Ramp Waveform"() -> (w586:i64[])
                n278 = local read "DNL_Ramp"() -> (w588:dbl[])
                n279 = local read "INL_Ramp"() -> (w587:dbl[])
                n280 = call-poly <vilib>:"Write To Spreadsheet File.vi"("delimiter (\\t)"=w581, "1D data"=string[] ["ADC Raw data", "DNL", "INL", "Histogram"], "file path (dialog if empty)"=w582) -> ("new file path (Not A Path if cancelled)"=w583:path)  [unwired: 5 in]
                n281 = Build Array(w586, w588, w587, w585) -> (w584:dbl[][])
                n282 = call-poly <vilib>:"Write To Spreadsheet File.vi"("delimiter (\\t)"=w581, "transpose? (no:F)"=w580, "append to file? (new file:F)"=w580, "2D data"=w584, "file path (dialog if empty)"=w583) -> ()  [unwired: 3 in, 1 out]
              }
            }
            "Ramp" <- 2 ("Select Tab")
          }
          frame "ADC Sine", Default {
            n283 = case shown="True" w590 {
              tunnel: w592 -> [_ w595]
              frame False {
              }
              frame True {
                n284 = Current VI's Path() -> (path=w596:path)
                n285 = call "Take fron panel screenshot.vi"("VI path"=w596, "Image path"=w595, "Visible area only? (f)"=FALSE, "File type (.jpg)"=enum16{".bmp", ".png", ".jpg"}.".png") -> ()  [unwired: 4 in, 1 out]
              }
            }
            n286 = case shown="True" w589 {
              tunnel: w593 -> [_ w604]
              frame False {
              }
              frame True {
                w600 = "," ("delimiter (\\t)")
                n287 = local read "Histogram Plot"() -> (w608:dbl[][])
                n288 = local read "Sine Waveform"() -> (w599:i64[])
                n289 = local read "DNL Plot"() -> (w611:dbl[])
                n290 = local read "INL Plot"() -> (w610:dbl[])
                n291 = Index Array(array=w608, index (row)=1 ("disabled index (col)")) -> (element=w607:dbl[])  [unwired: 1 in]
                n292 = call-poly <vilib>:"Write To Spreadsheet File.vi"("delimiter (\\t)"=w600, "1D data"=string[] ["DNL", "INL", "Histogram", "Rawdata"], "file path (dialog if empty)"=w604) -> ("new file path (Not A Path if cancelled)"=w603:path)  [unwired: 5 in]
                n293 = Build Array(w611, w610, w607, w599) -> (w609:dbl[][])
                n294 = call-poly <vilib>:"Write To Spreadsheet File.vi"("delimiter (\\t)"=w600, "transpose? (no:F)"=TRUE, "append to file? (new file:F)"=TRUE, "2D data"=w609, "file path (dialog if empty)"=w603) -> ()  [unwired: 3 in, 1 out]
              }
            }
            n295 = local write "Main Tab"(4) -> ()
            "Sine" <- 1
          }
          frame "SNR" {
            n296 = case shown="True" w613 {
              tunnel: w616 -> [_ w618]
              frame False {
              }
              frame True {
                n297 = Current VI's Path() -> (path=w619:path)
